vi "OpenAndSendDataToSubVi(SubVI).vi"(0 "reference":refnum<vi>, 1 "Control Name":string, 2 "element":T1={"main stm"=enum."idle", "STM Graph"={"Graph settings"={"Axis X Min"=0.0, "Axis X Name"="", "Axis X Max"=1.0, "Axis Y Min"=0.0, " Axis Y Name"="", "Axis Y Max"=1.0, "Autoscale"=enum."Yes", "Choice Line"=0.0}, "Lines"=[], "Data"=""}} {"STM Graph"."Lines"."Color" format="%x"}) -> ()   [LabVIEW 2018]
uses:
  Windows/Settings/GraphSettings/GraphSettings_STM.ctl
  Windows/Settings/GraphSettings/GraphSettings_ITEM.ctl
  CTL/STM GRAPH.ctl
  CTL/Graph settings.ctl
  CTL/Line.ctl
  Windows/Settings/View.ctl
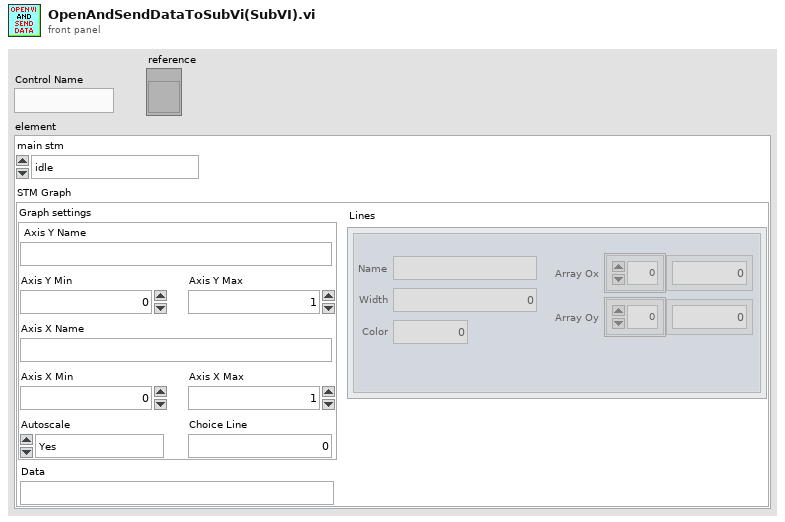
[diagram p1: front panel]
types:
  T1 = typedef "GraphSettings_STM.ctl" = cluster{"main stm":T2, "STM Graph":T3}
  T2 = typedef "GraphSettings_ITEM.ctl" = enum16{"idle", "init", "close", "_____ SETTINGS _____ ", "Receive Data", "Send Data", "Change Line", "Delete Line", "Add Line", "FrontPanelWindowState", "Change Color", "Choice Line"}
  T3 = typedef "STM GRAPH.ctl" = cluster{"Graph settings":T4, "Lines":T5[], "Data":string}
  T4 = typedef "Graph settings.ctl" = cluster{"Axis X Min":dbl, "Axis X Name":string, "Axis X Max":dbl, "Axis Y Min":dbl, " Axis Y Name":string, "Axis Y Max":dbl, "Autoscale":enum16{"Yes", "No", "Only Oy", "Only Ox"}, "Choice Line":dbl}
  T5 = typedef "Line.ctl" = cluster{"Width":dbl, "Color":i64, "Array Oy":dbl[], "Array Ox":dbl[], "Name":string, "Plot Visible":T6}
  T6 = typedef "View.ctl" = bool
  T7 = enum32{"Invalid", "Default", "Floating", "Floating/Auto-Hide", "Modal"}
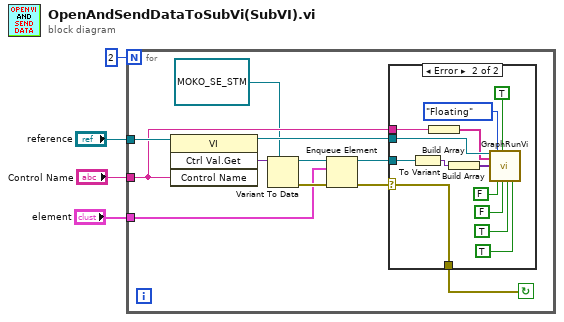
[diagram p0: block diagram]
diagram:
  n1 = for {
    N: 2 -> [_]
    tunnel: "reference" -> [w9]
    tunnel: "Control Name" -> [w8]
    tunnel: "element" -> [w5]
    stop <- w10 continue-if-true
    n2 = invoke on="Invoke Node" class="VI" method="Ctrl Val.Get"(reference=w9, "Control Name"=w8) -> (reference out=w14:refnum<vi>, "Get Control Value Variant"=w15:variant)  [unwired: 2 in, 2 out]
    n3 = Variant To Data(type=refnum<queue> refnum ("queue in"), Variant=w15) -> (data=w6:refnum<queue>, error out=w13:errorcluster)  [unwired: 1 in]
    n4 = Enqueue Element(queue=w6, element=w5, error in (no error)=w13) -> (queue out=w12:refnum<queue>, error out=w11:errorcluster)  [unwired: 1 in, 1 out]
    n5 = case shown="Error" w11 {
      selector: w11 -> [w16 w19]
      tunnel: w14 -> [_ w27]
      tunnel: w12 -> [_ w20]
      tunnel: [w16 w19] -> w10
      tunnel: w8 -> [_ w18]
      frame No Error {
      }
      frame Error {
        n6 = To Variant(anything=w20) -> (Variant=w29:variant)
        n7 = Build Array(w18) -> (w17:string[])
        n8 = Build Array(w29) -> (w28:variant[])
        n9 = call "GraphRunVi.vi"("VI Refnum"=w27, "Controls Name"=w17, "Values"=w28, "Front Panel Behavior"=T7."Floating", "Wait Until Done"=FALSE, "ShowFP"=TRUE, "LoadVariableIf RUN"=FALSE, "DoNotCentered If RUN"=TRUE, "Front Panel Window:Is Frontmost"=TRUE) -> ()  [unwired: 10 in, 1 out]
      }
    }
  }
